vi "LABVIEW_robot_control.vi"() -> ()   [LabVIEW 2014]
doc: "This example performs writes and reads on a serial port, as directed by the user. You can press the Write and Read buttons, and change the Read Count, while the example is running.\n\nThe parameters set for the serial port must match the parameters of the connected instrument or device. In this example, the Read Count parameter specifies the number of bytes that the serial port reads. If there were more bytes at the port than the specified number, those bytes would not be read. If there were less bytes at the port than the specified number, you would receive a timeout error.\n\nThis example expands upon the flow control options for XON and XOFF, allowing the user to choose those control characters. Also, the user can enable or disable a termination character. Some devices require a termination character in order to identify the end of command strings. Some devices send a termination character to signify the end of data to be read. This example shows how you can end the Read operation once a termination character is detected in the buffer and/or append a termination character at the end of the Write data."
uses:
  <vilib>/Instr/_visa.llb/VISA Configure Serial Port (Instr).vi
panel:
  in  "stop bits (10: 1 bit)":u16(ring)=10 items=["1.0"=10, "1.5"=15, "2.0"=20]
  in  "parity (0:none)":enum16{"None", "Odd", "Even", "Mark", "Space"}(ring)
  in  "data bits (8)":u16=8 min=5 max=8 step=1
  in  "baud rate (9600)":u32=9600
  in  "STOP":bool
  in  "RIGHT":bool
  in  "LEFT":bool
  in  "REVERSE":bool
  in  "Stop":bool
  in  "FORWARD":bool
  in  "VISA resource name":refnum<visa-resource-name>="COM1"
  # "Overview: Demonstrates the use of the VISA functions to write commands to and read responses from a serial instrument continuously in a loop.\nRequirements: NI-VISA Driver\nInstructions:\n1. Run the VI.\n2. Specify a Command and click the Write button.\n3. Read a Response by clicking the Read button.\n4. Click Stop to stop the VI."
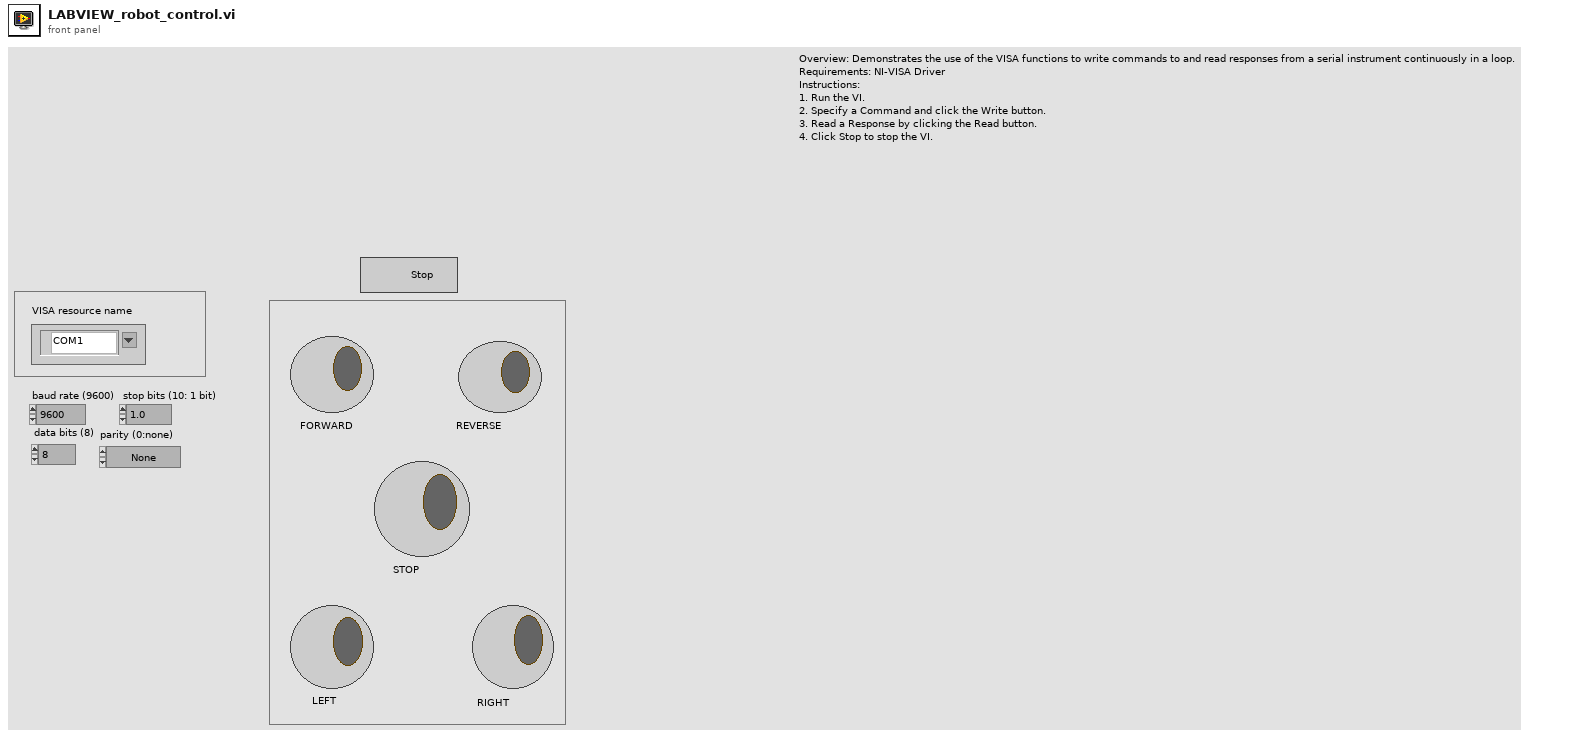
[diagram p1: front panel]
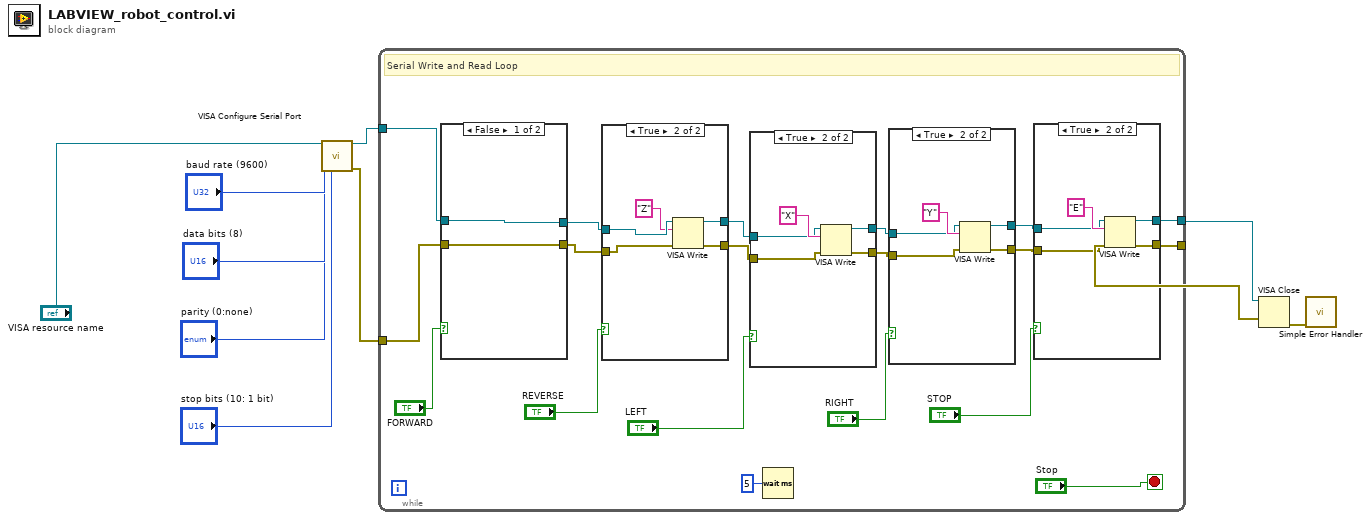
[diagram p0: block diagram]
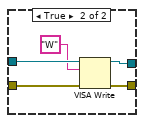
[diagram p6: hidden frame]
diagram:
  n1 = call-poly "VISA Configure Serial Port"("VISA resource name"="VISA resource name", "baud rate (9600)"="baud rate (9600)", "data bits (8)"="data bits (8)", "parity (0:none)"="parity (0:none)", "stop bits (10: 1 bit)"="stop bits (10: 1 bit)") -> ("VISA resource name out"=w7:refnum<visa-resource-name>, "error out"=w8:errorcluster)  [unwired: 5 in, 4 out]
  n2 = while {
    tunnel: w8 -> [w28]
    tunnel: w7 -> [w25]
    tunnel: [w16] -> w6
    tunnel: [w17] -> w5
    stop <- "Stop" stop-if-true
    # "Serial Write and Read Loop"
    n3 = case shown="False" "FORWARD" {
      tunnel: w25 -> [w59 w64]
      tunnel: w28 -> [w58 w63]
      tunnel: [w59 w62] -> w26
      tunnel: [w58 w61] -> w27
      frame False {
      }
      frame True {
        n4 = VISA Write(VISA resource name=w64, write buffer="W", error in (no error)=w63) -> (VISA resource name out=w62:refnum<visa-resource-name>, error out=w61:errorcluster)  [unwired: 1 out]
      }
    }
    n5 = case shown="True" "REVERSE" {
      tunnel: [w52 w57] -> w23
      tunnel: [w51 w56] -> w22
      tunnel: w27 -> [w51 w55]
      tunnel: w26 -> [w52 w54]
      frame False {
      }
      frame True {
        n6 = VISA Write(VISA resource name=w54, write buffer="Z", error in (no error)=w55) -> (VISA resource name out=w57:refnum<visa-resource-name>, error out=w56:errorcluster)  [unwired: 1 out]
      }
    }
    n7 = case shown="True" "LEFT" {
      tunnel: [w45 w50] -> w21
      tunnel: [w44 w49] -> w20
      tunnel: w22 -> [w44 w46]
      tunnel: w23 -> [w45 w47]
      frame False {
      }
      frame True {
        n8 = VISA Write(VISA resource name=w47, write buffer="X", error in (no error)=w46) -> (VISA resource name out=w50:refnum<visa-resource-name>, error out=w49:errorcluster)  [unwired: 1 out]
      }
    }
    n9 = Wait (ms)(milliseconds to wait=u32 5) -> ()  [unwired: 1 out]
    n10 = case shown="True" "RIGHT" {
      tunnel: [w38 w43] -> w19
      tunnel: [w37 w42] -> w18
      tunnel: w20 -> [w37 w39]
      tunnel: w21 -> [w38 w40]
      frame False {
      }
      frame True {
        n11 = VISA Write(VISA resource name=w40, write buffer="Y", error in (no error)=w39) -> (VISA resource name out=w43:refnum<visa-resource-name>, error out=w42:errorcluster)  [unwired: 1 out]
      }
    }
    n12 = case shown="True" "STOP" {
      tunnel: [w31 w36] -> w17
      tunnel: [w30 w35] -> w16
      tunnel: w18 -> [w30 w32]
      tunnel: w19 -> [w31 w33]
      frame False {
      }
      frame True {
        n13 = VISA Write(VISA resource name=w33, write buffer="E", error in (no error)=w32) -> (VISA resource name out=w36:refnum<visa-resource-name>, error out=w35:errorcluster)  [unwired: 1 out]
      }
    }
  }
  n14 = VISA Close(VISA resource name=w5, error in (no error)=w6) -> (error out=w9:errorcluster)
  n15 = call <vilib>:"Simple Error Handler.vi"("error in (no error)"=w9) -> ()  [unwired: 1 in, 8 out]
